vi "LoggingData.vi"(8 "error in (no error)":errorcluster, 10 "Start time":u32, 11 "Refmum":refnum<file>) -> (0 "error out":errorcluster, 3 "Byte Stream File out":refnum<file>)   [LabVIEW 2017]
uses:
  Framework/Robot Global Data.vi
  Drive/Implementation/Drive Published Globals.vi
  <vilib>/NI_Real-Time Target Support.lvlib
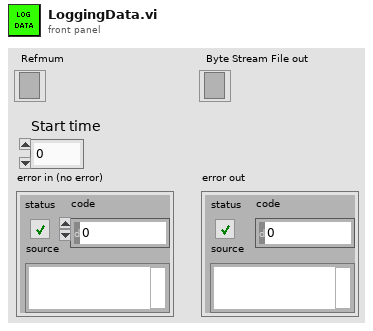
[diagram p1: front panel]
types:
  T1 = typedef "WPI_DriverStationRobotMode2.ctl" = enum16{"Autonomous Disabled", "Autonomous Enabled", "Teleop Disabled", "Teleop Enabled", "Disconnected", "Finish", "Test Disabled", "Test Enabled", "Emergency Stopped"}
  T2 = typedef "NI_Real-Time Target Support.lvlib/RT CPU Load.ctl" = cluster{"Total (%)":dbl, "Time Critical (%)":dbl, "Timed Structures (%)":dbl, "High (%)":dbl, "Above Normal (%)":dbl, "Normal (%)":dbl, "Background (%)":dbl, "Idle (%)":dbl, "ISR (%)":dbl}
  T3 = cluster{"Yaw":dbl, "Roll":dbl, "Pitch":dbl, "Heading":dbl, "Fused Heading":dbl}
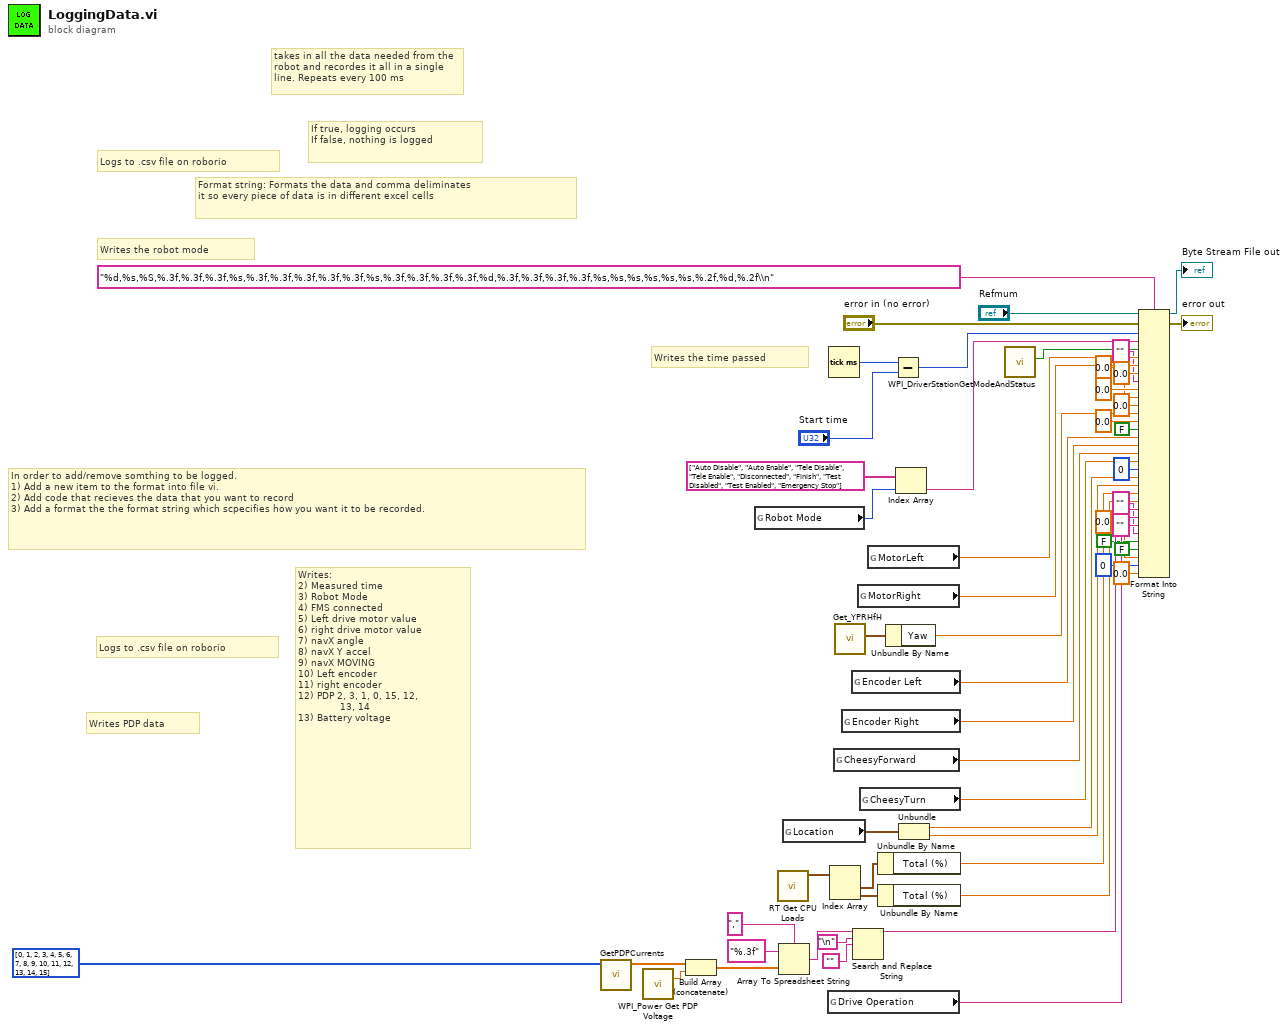
[diagram p0: block diagram]
diagram:
  # "Writes the time passed"
  # "Writes PDP data"
  # "Writes the robot mode"
  # "Logs to .csv file on roborio"
  # "Format string: Formats the data and comma deliminates \nit so every piece of data is in different excel cells"
  # "In order to add/remove somthing to be logged.\n1) Add a new item to the format into file vi.\n2) Add code that recieves the data that you want to record\n3) Add a format the the format string which scpecifies how you want it to be recorded."
  # "Logs to .csv file on roborio"
  # "If true, logging occurs\nIf false, nothing is logged"
  # "Writes:\n2) Measured time\n3) Robot Mode\n4) FMS connected\n5) Left drive motor value\n6) right drive motor value\n7) navX angle\n8) navX Y accel\n9) navX MOVING\n10) Left encoder\n11) right encoder\n12) PDP 2, 3, 1, 0, 15, 12,\n              13, 14\n13) Battery voltage"
  # "takes in all the data needed from the robot and recordes it all in a single line. Repeats every 100 ms"
  n1 = call "GetPDPCurrents.vi"("Channels"=i32[] [0, 1, 2, 3, 4, 5, 6, 7, 8, 9, 10, 11, 12, 13, 14, 15]) -> ("Currents"=w50:dbl[])  [unwired: 10 in]
  n2 = call <vilib>:"WPI_Power Get PDP Voltage.vi"() -> ("voltage (V)"=w48:dbl)  [unwired: 14 in, 1 out]
  n3 = Build Array (concatenate)(w50, w48) -> (w51:dbl[])
  n4 = global read "Robot Global Data.vi" "Robot Mode"() -> (w40:T1)
  n5 = call <vilib>:"RT Get CPU Loads.vi"() -> ("CPU loads"=w43:T2[])  [unwired: 10 in, 1 out]
  n6 = Array To Spreadsheet String(delimiter (Tab)=",", array=w51, 3:"%.3f" ("format string")) -> (spreadsheet string=w18:string)
  n7 = global read "Drive Published Globals.vi" "Location"() -> (w39:cluster{dbl, dbl})
  n8 = global read "Robot Global Data.vi" "Drive Operation"() -> (w20:string)
  n9 = Tick Count (ms)() -> (millisecond timer value=w37:u32)
  n10 = Index Array(array=w43) -> (element #1=w45:T2, element #2=w44:T2)  [unwired: 2 in]
  n11 = global read "Robot Global Data.vi" "CheesyForward"() -> (w24:dbl)
  n12 = call <vilib>:"Get_YPRHfH.vi"() -> ("YRPHfH"=w35:T3)  [unwired: 11 in]
  n13 = global read "Drive Published Globals.vi" "Encoder Right"() -> (w23:dbl)
  n14 = global read "Drive Published Globals.vi" "Encoder Left"() -> (w22:dbl)
  n15 = Search and Replace String(input string=w18, search string="\n", replace string="") -> (result string=w16:string)  [unwired: 5 in, 3 out]
  n16 = global read "Drive Published Globals.vi" "MotorRight"() -> (w30:dbl)
  n17 = global read "Robot Global Data.vi" "CheesyTurn"() -> (w25:dbl)
  n18 = global read "Drive Published Globals.vi" "MotorLeft"() -> (w32:dbl)
  n19 = Unbundle By Name(w45) -> ("Total (%)"=w28:dbl)
  n20 = Unbundle By Name(w44) -> ("Total (%)"=w29:dbl)
  n21 = Unbundle By Name(w35) -> ("Yaw"=w21:dbl)
  n22 = Subtract(x=w37, y="Start time") -> (x-y=w38:u32)
  n23 = Index Array(array=string[] ["Auto Disable", "Auto Enable", "Tele Disable", "Tele Enable", "Disconnected", "Finish", "Test Disabled", "Test Enabled", "Emergency Stop"], index=w40) -> (element=w42:string)
  n24 = Unbundle(w39) -> (w26:dbl, w27:dbl)
  n25 = call <vilib>:"WPI_DriverStationGetModeAndStatus.vi"() -> ("FMS Attached"=w34:bool)  [unwired: 10 in, 1 out]
  n26 = Format Into String(format string="%d,%s,%S,%.3f,%.3f,%.3f,%s,%.3f,%.3f,%.3f,%.3f,%.3f,%s,%.3f,%.3f,%.3f,%.3f,%d,%.3f,%.3f,%.3f,%.3f,%s,%s,%s,%s,%s,%s,%.2f,%d,%.2f\\n", initial string="Refmum", error in="error in (no error)", w38, w42, w34, w32, w30, 0.0 ("input 6"), "" ("input 7"), 0.0 ("input 8"), 0.0 ("input 9"), 0.0 ("input 10"), w21, 0.0 ("input 12"), FALSE ("input 13"), w22, w23, w24, w25, u32 0 ("input 18"), w26, w27, w28, w29, w16, w20, "" ("input 25"), "" ("input 26"), FALSE ("input 27"), FALSE ("input 28"), 0.0 ("input 29"), 0 ("input 30"), 0.0 ("input 31")) -> (resulting string=→"Byte Stream File out":refnum<file>, error out=→"error out":errorcluster)
